vi "Read Severity Code.vi"(8 "error in (no error)":errorcluster, 11 "abs_EventLog in":refnum<class "abs_EventLog.lvclass">) -> (0 "error out":errorcluster, 2 "Severity Code":T1=enum."error", 3 "abs_EventLog out":refnum<class "abs_EventLog.lvclass">)   [LabVIEW 2021, in "abs_EventLog.lvclass"]
uses:
  abs_EventLog.lvclass
  Support/Severity Code.ctl
  abs_EventLog.lvclass/abs_EventLog.ctl
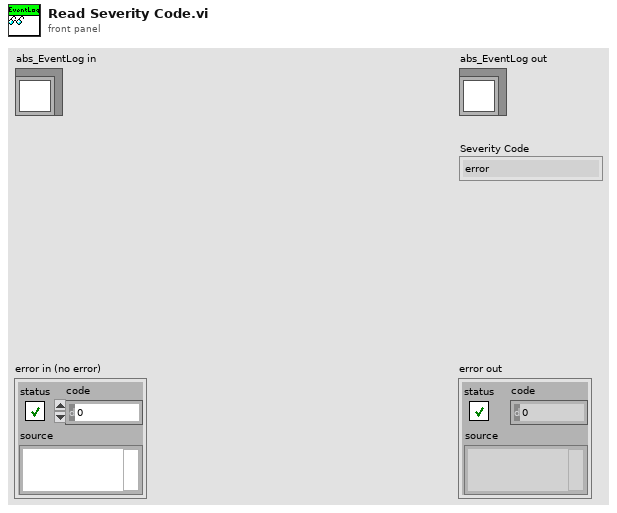
[diagram p1: front panel]
types:
  T1 = typedef "abs_EventLog.lvclass/Severity Code.ctl" = enum16{"emergency", "alert", "critical", "error", "warning", "notice", "info", "debug"}
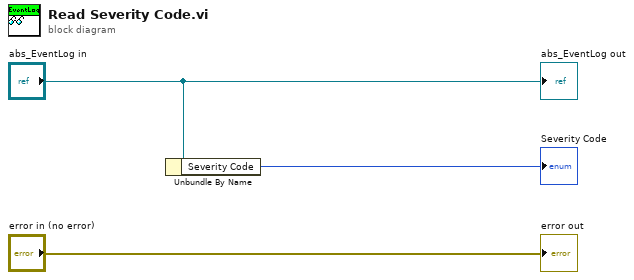
[diagram p0: block diagram]
diagram:
  n1 = Unbundle By Name("abs_EventLog in") -> ("Severity Code"=→"Severity Code":T1)
  "error out" <- "error in (no error)"
  "abs_EventLog out" <- "abs_EventLog in"
